vi "Remove first row.vi"(1 "Data with comments\nin first row":sgl[][](array[numeric]) format="%.2f") -> (0 "The same data\nwithout first raw":sgl[][](array[numeric]) format="%.2f")   [LabVIEW 2010]
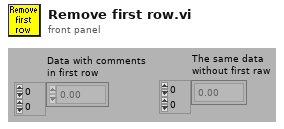
[diagram p1: front panel]
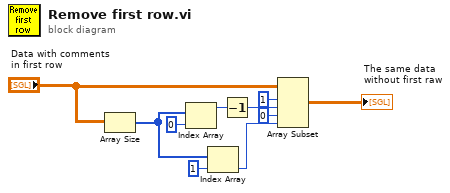
[diagram p0: block diagram]
diagram:
  n1 = Array Size(array="Data with comments\nin first row") -> (size(s)=w6:i32[])
  n2 = Index Array(array=w6, index=0 ("Index")) -> (element=w9:i32)
  n3 = Index Array(array=w6, index=1 ("Index")) -> (element=w10:i32)
  n4 = Decrement(x=w9) -> (x-1=w1:i32)
  n5 = Array Subset(array="Data with comments\nin first row", index (row)=1 ("Array Index"), length (row)=w1, index (col)=0 ("Array Index"), length (col)=w10) -> (→"The same data\nwithout first raw":sgl[][])
